vi "CryoServer Read Line.vi"(8 "error in (no error)":errorcluster, 10 "timeout ms (5000)":i32=5000, 11 "connection ID":refnum<k5>) -> (0 "error out":errorcluster, 2 "data out":string, 3 "connection ID out":refnum<k5>)   [LabVIEW 2021, in "CryoServer.lvclass"]
uses:
  CryoServer.lvclass
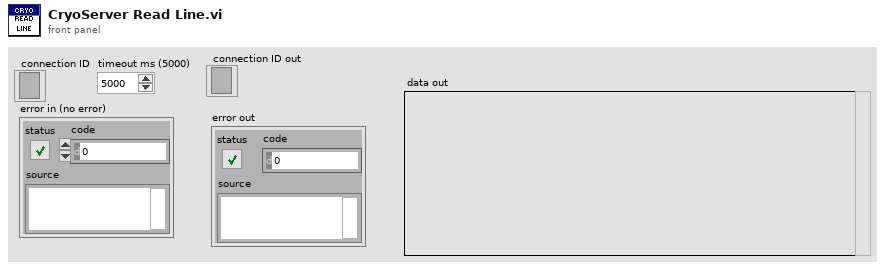
[diagram p1: front panel]
types:
  T1 = enum16{"Standard", "Buffered", "CRLF", "Immediate"}
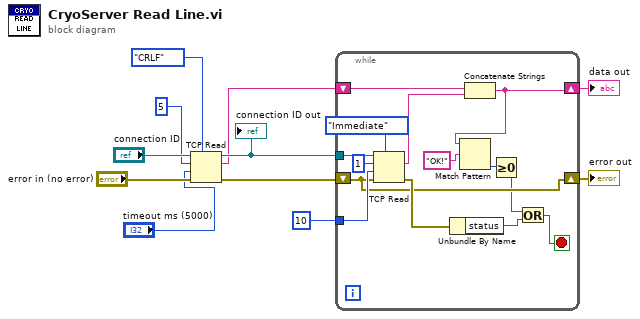
[diagram p0: block diagram]
diagram:
  n1 = TCP Read(connection ID="connection ID", bytes to read=5, error in (no error)="error in (no error)", 7:T1."CRLF" ("mode (standard)"), 9:"timeout ms (5000)") -> (connection ID out=w10:refnum<k5>, data out=w9:string, error out=w11:errorcluster)
  "connection ID out" <- w10
  n2 = while {
    tunnel: w10 -> [w25]
    shift-right: [w12] -> w6
    shift-left: w9 -> [w21]
    shift-right: [w17] -> w2
    shift-left: w11 -> [w17]
    tunnel: 10 ("timeout ms (25000)") -> [w18]
    stop <- w22 stop-if-true
    n3 = TCP Read(connection ID=w25, bytes to read=1, error in (no error)=w17, 7:T1."Immediate" ("mode (standard)"), 9:w18) -> (data out=w19:string, error out=w20:errorcluster)  [unwired: 1 out]
    n4 = Unbundle By Name(w20) -> ("status"=w23:bool)
    n5 = Concatenate Strings(w21, w19) -> (w12:string)
    n6 = Match Pattern(string=w12, regular expression="OK!") -> (offset past match=w15:i32)  [unwired: 1 in, 3 out]
    n7 = Greater Or Equal To 0?(x=w15) -> (x >= 0?=w14:bool)
    n8 = Or(x=w14, y=w23) -> (x .or. y?=w22:bool)
  }
  "data out" <- w6
  "error out" <- w2
